vi "MB Ethernet Slave PLC.vi"() -> ()   [LabVIEW 2017]
uses:
  NI Modbus.llb/MB Slave Init (poly).vi
  NI Modbus.llb/MB Globals.vi
  NI Modbus.llb/MB Slave Read All Coils (poly).vi
  NI Modbus.llb/MB Slave Read All Holding Registers (poly).vi
  NI Modbus.llb/MB Slave Write Holding Registers (poly).vi
  NI Modbus.llb/MB Slave Write Discrete Inputs (poly).vi
panel:
  in  "Discrete Inputs (Master can only read these)":bool[](array[boolean])=[FALSE, FALSE, FALSE, FALSE]
  out "Consumo eléctrico Isla Numblar":u16[](array[numeric])
  in  "Listening Port":u16=502
  in  "Stop":bool
  out "Holding Registers":u16[](array[numeric]) caption="Holding Registers (Master can write in these registers)"
  out "Coils":bool[](array[boolean]) caption="Coils (Master can write coils)"
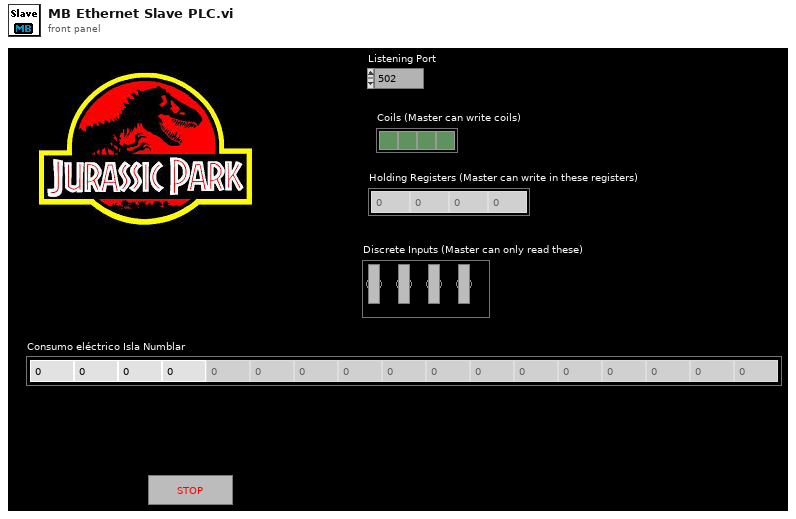
[diagram p1: front panel]
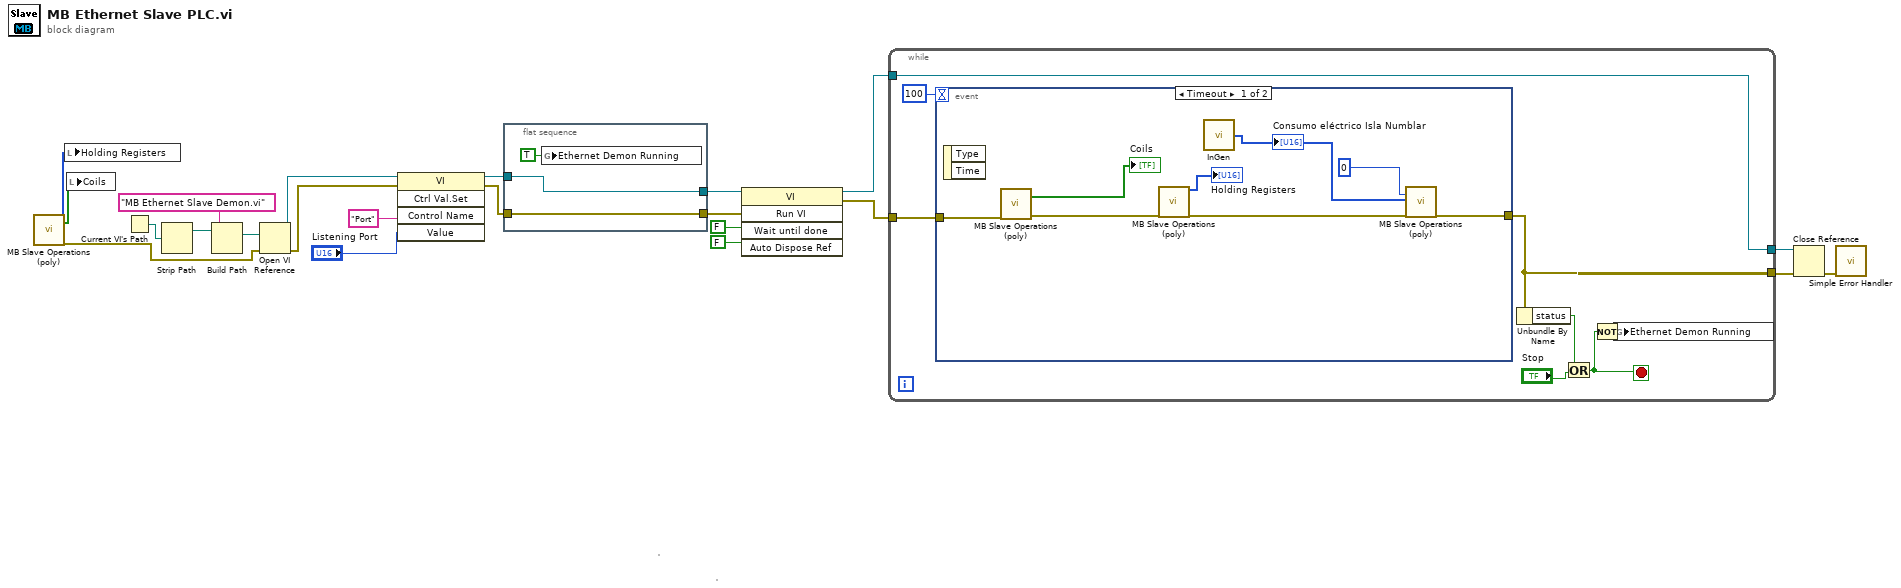
[diagram p0: block diagram]
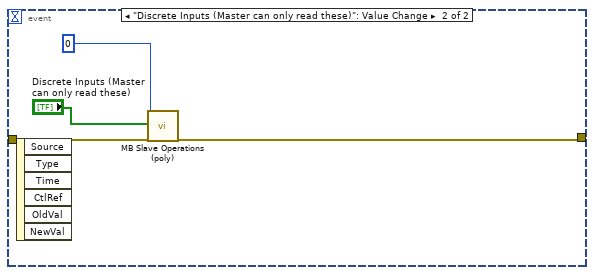
[diagram p2: hidden frame]
diagram:
  n1 = call-poly "MB Slave Operations (poly).vi"() -> ("Holding Registers"=w22:u16[], "Coils"=w5:bool[], "error out"=w8:errorcluster)  [unwired: 1 in, 16 out]
  n2 = local write "Holding Registers"(w22) -> ()
  n3 = local write "Coils"(w5) -> ()
  n4 = Current VI's Path() -> (path=w18:path)
  n5 = Strip Path(path=w18) -> (stripped path=w19:path)  [unwired: 1 out]
  n6 = Build Path(base path=w19, name or relative path="MB Ethernet Slave Demon.vi") -> (appended path=w21:path)
  n7 = Open VI Reference(vi path=w21, error in (no error)=w8) -> (vi reference=w15:refnum<vi>, error out=w14:errorcluster)  [unwired: 4 out]
  n8 = invoke class="VI" method="Ctrl Val.Set"(reference=w15, error in=w14, "Control Name"="Port", "Value"="Listening Port") -> (reference out=w1:refnum<vi>, error out=w2:errorcluster)  [unwired: 1 in, 3 out]
  n9 = flat-sequence {
    tunnel: [w25] -> w7
    tunnel: w2 -> [w25]
    tunnel: [w23] -> w4
    tunnel: w1 -> [w23]
    frame #0 {
      n10 = global write "MB Globals.vi" "Ethernet Demon Running"(TRUE ("Slave Demon Running")) -> ()
    }
  }
  n11 = invoke class="VI" method="Run VI"(reference=w4, error in=w7, "Wait until done"=FALSE, "Auto Dispose Ref"=FALSE) -> (reference out=w10:refnum<vi>, error out=w6:errorcluster)  [unwired: 1 in, 3 out]
  n12 = while {
    tunnel: [w28] -> w11
    tunnel: w10 -> [w28]
    tunnel: [w27] -> w9
    tunnel: w6 -> [w26]
    stop <- w29 stop-if-true
    n13 = event shown="[0] Timeout" {
      selector: _ -> [_ _]
      dyn-events: _ -> [_ _]
      timeout: 100 -> [_ _]
      tunnel: w26 -> [w41 w45]
      tunnel: [w36 w42] -> w27
      event Timeout {
        n14 = event-data() -> ()  [unwired: 3 out]
        n15 = call-poly "MB Slave Operations (poly).vi"("error in"=w41) -> ("Coils"=→"Coils":bool[], "error out"=w39:errorcluster)  [unwired: 17 out]
        n16 = call-poly "MB Slave Operations (poly).vi"("error in"=w39) -> ("Holding Registers"=→"Holding Registers":u16[], "error out"=w35:errorcluster)  [unwired: 17 out]
        n17 = call "InGen.vi"() -> ("Variables de planta"=w34:u16[])
        "Consumo eléctrico Isla Numblar" <- w34
        n18 = call-poly "MB Slave Operations (poly).vi"("Starting Address"=u16 0 ("Address"), "Holding Registers"=w34, "error in"=w35) -> ("error out"=w36:errorcluster)  [unwired: 1 in, 15 out]
      }
      event "Discrete Inputs (Master can only read these)": Value Change {
        n19 = event-data() -> ()  [unwired: 7 out]
        n20 = call-poly "MB Slave Operations (poly).vi"("Starting Address"=u16 0, "Discrete Inputs"="Discrete Inputs (Master can only read these)", "error in"=w45) -> ("error out"=w42:errorcluster)  [unwired: 1 in, 15 out]
      }
    }
    n21 = Unbundle By Name(w27) -> ("status"=w32:bool)
    n22 = Or(x=w32, y="Stop") -> (x .or. y?=w29:bool)
    n23 = Not(x=w29) -> (.not. x?=w30:bool)
    n24 = global write "MB Globals.vi" "Ethernet Demon Running"(w30) -> ()
  }
  n25 = Close Reference(reference=w11, error in (no error)=w9) -> (error out=w3:errorcluster)
  n26 = call <vilib>:"Simple Error Handler.vi"("error in (no error)"=w3) -> ()  [unwired: 1 in, 8 out]
